vi "Write Result Channel GUID.vi"(8 "error in (no error)":errorcluster, 10 "Result Channel GUID":string, 11 "WaveformCalculation in":refnum<class "WaveformCalculation.lvclass">) -> (0 "error out":errorcluster, 3 "WaveformCalculation out":refnum<class "WaveformCalculation.lvclass">)   [LabVIEW 2015, in "WaveformCalculation.lvclass"]
uses:
  WaveformCalculation.lvclass
  WaveformCalculation.lvclass/WaveformCalculation.ctl
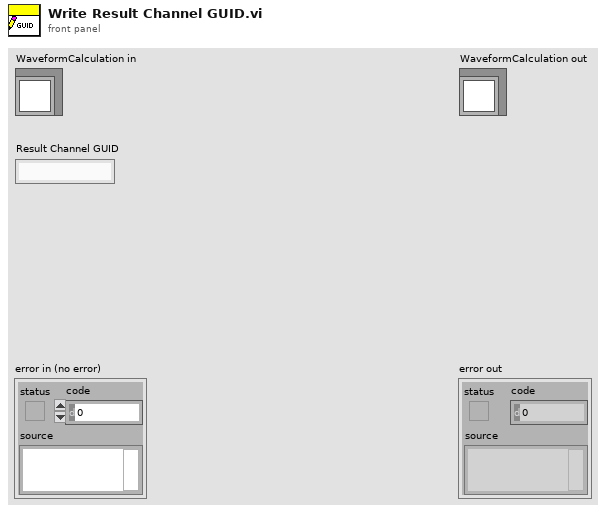
[diagram p1: front panel]
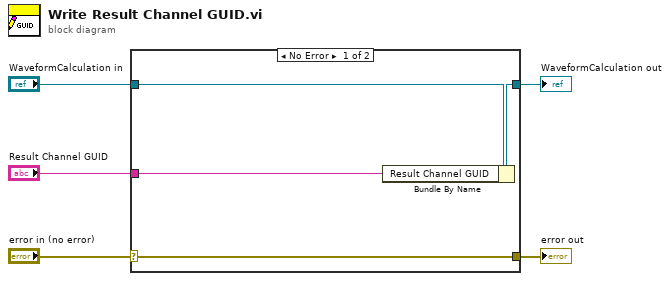
[diagram p0: block diagram]
diagram:
  n1 = case shown="No Error" "error in (no error)" {
    selector: "error in (no error)" -> [w9 w10]
    tunnel: [w9 w10] -> w4
    tunnel: [w7 w11] -> w2
    tunnel: "WaveformCalculation in" -> [w8 w11]
    tunnel: "Result Channel GUID" -> [w6 _]
    frame No Error {
      n2 = Bundle By Name(cluster=w8, "Result Channel GUID"=w6) -> (w7:refnum<class "WaveformCalculation.lvclass">)
    }
    frame Error {
    }
  }
  "error out" <- w4
  "WaveformCalculation out" <- w2
